vi "Configure Multitone Export File.vi"(5 "Number Of Bits (0)":i32, 6 "Dither (0: dgNoDither)":i32(ring) items=["dgNoDither", "dgTriangular", "dgRectangular"], 7 "File Name (\"MyFile.arb\")":string="\"MyFile.arb\"", 8 "error in (no error)":errorcluster, 9 "Mode (0: mtArbFile)":i32(ring) items=["mtArbFile", "mtWavFile"], 10 "Channel (0: A)":i32(ring) items=["A", "B"], 11 "VISA resource name":refnum<visa-resource-name>) -> (0 "error out":errorcluster, 3 "VISA resource name out":refnum<visa-resource-name>)   [LabVIEW 2014, in "Stanford Research SR1.lvlib"]
doc: "Exports the multitone waveformto either an arbitrary waveformor a .WAVfile with the specified filename, bit resolution and dither options."
uses:
  Stanford Research SR1.lvlib
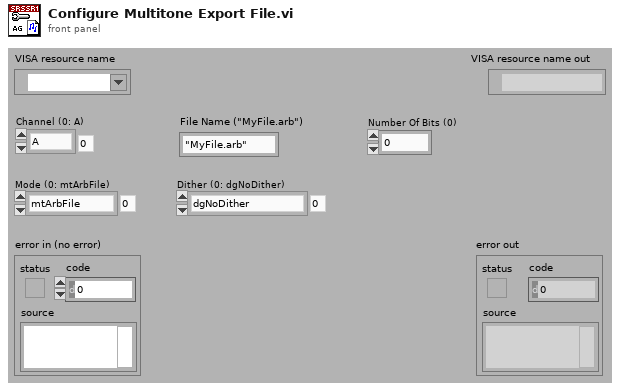
[diagram p1: front panel]
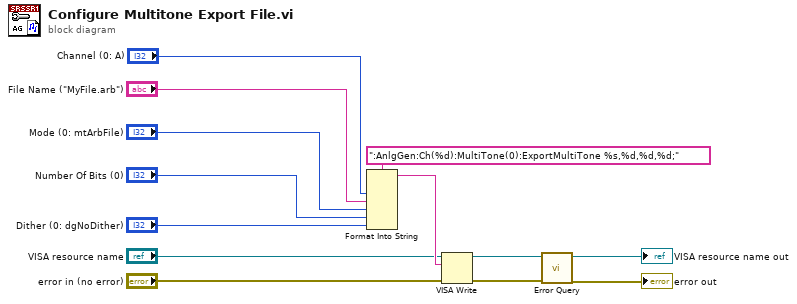
[diagram p0: block diagram]
diagram:
  n1 = Format Into String(format string=":AnlgGen:Ch(%d):MultiTone(0):ExportMultiTone %s,%d,%d,%d;", "Channel (0: A)", "File Name (\"MyFile.arb\")", "Mode (0: mtArbFile)", "Number Of Bits (0)", "Dither (0: dgNoDither)") -> (resulting string=w12:string)  [unwired: 2 in, 1 out]
  n2 = VISA Write(VISA resource name="VISA resource name", write buffer=w12, error in (no error)="error in (no error)") -> (VISA resource name out=w9:refnum<visa-resource-name>, error out=w8:errorcluster)  [unwired: 1 out]
  n3 = call "Error Query.vi"("error in (no error)"=w8, "VISA resource name"=w9) -> ("error out"=→"error out":errorcluster, "VISA resource name out"=→"VISA resource name out":refnum<visa-resource-name>)  [unwired: 6 in, 2 out]
